vi "Hokuyo URG Series Configure and Acquire Data.vi"() -> ()   [LabVIEW 2011]
doc: "This example shows how to configure the URG to aquire data and then creates a polar graph using the magnitude and direction arrays.\n\nTo use this example with a USB LIDAR on a cRIO target, change the VISA resource name type to USB Raw. See the help for the control for additional information."
uses:
  Public/Initialize-Standard.vi
  Hokuyo URG Series.lvlib
panel:
  in  "Encoding Width":u16(ring)=3 items=["2 Byte"=2, "3 Byte"=3]
  in  "Max (m)":dbl=4.1
  in  "Plot Color":u32(colorbox)=6618880
  in  "Grid Color":u32(colorbox)=16777222
  in  "Protocol":u32(ring)=2 items=["Convert to Latest", "SCIP 1.1", "SCIP 2.0"]
  in  "ID Query?":bool=TRUE
  in  "Cluster Count":dbl=1.0
  in  "Start Point":dbl=-120.0
  in  "End Point":dbl=120.0
  in  "Checksum":bool
  in  "VISA resource name":refnum<visa-resource-name>
  in  "Stop":bool
  in  "polar attributes (hidden)":T1={"maximum"=30000.0, "minimum"=0.0, "clip to min"=FALSE, "log?(F)"=TRUE, "grid color"=6710886, "plot color"=65280, "fmt and prec"={"format"=enum."Decimal", "precision"=0}, "visible section"=8} {"minimum" format="%0.2f"; "maximum" format="%0.2f"}
  out "Data Aquired":picture
  # "(c) 2009 National Instruments.  ALL RIGHTS RESERVED."
  # "Instrument Configuration"
  # "Measurement Configuration"
  # "Plot Display Configuration"
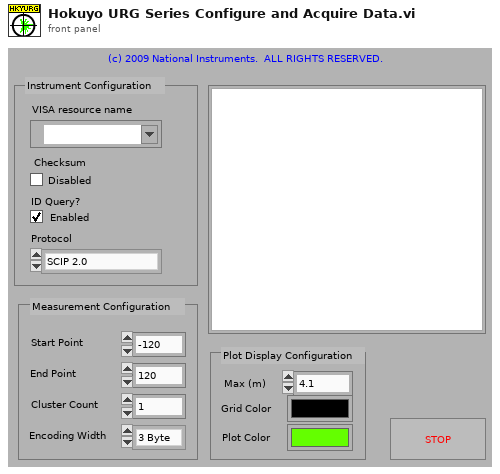
[diagram p1: front panel]
types:
  T1 = cluster{"maximum":dbl, "minimum":dbl, "clip to min":bool, "log?(F)":bool, "grid color":u32, "plot color":u32, "fmt and prec":cluster{"format":enum8{"Decimal", "Scientific", "Engineering", "Binary", "Octal", "Hex"}, "precision":u8}, "visible section":u16}
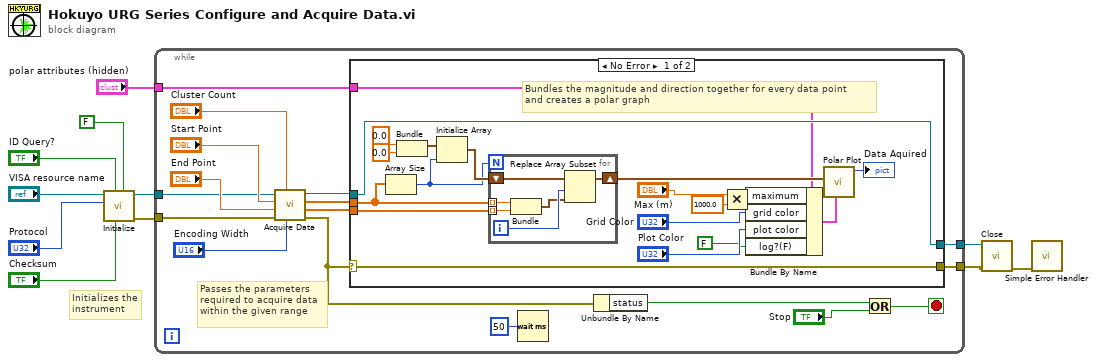
[diagram p0: block diagram]
diagram:
  # "Initializes the instrument"
  n1 = call-poly "Initialize.vi"("Reset? (F: No)"=FALSE ("Reset Instrument (Disabled)"), "Checksum (Disabled)"="Checksum", "ID Query? (Enabled)"="ID Query?", "Protocol (2: SCIP 2.0)"="Protocol", "VISA resource name"="VISA resource name") -> ("error out"=w2:errorcluster, "VISA resource name out"=w3:refnum<visa-resource-name>)  [unwired: 5 in]
  n2 = while {
    tunnel: w3 -> [w16]
    tunnel: [w28] -> w11
    tunnel: [w27] -> w4
    tunnel: w2 -> [w15]
    tunnel: "polar attributes (hidden)" -> [w14]
    stop <- w24 stop-if-true
    # "Passes the parameters\nrequired to acquire data\nwithin the given range"
    n3 = call "Acquire Data.vi"("Data Encoding Width (3 Byte)"="Encoding Width", "Cluster Count (1)"="Cluster Count", "error in (no error)"=w15, "End Point (120°)"="End Point", "Start Point (-120°)"="Start Point", "VISA resource name"=w16) -> ("error out"=w20:errorcluster, "Direction"=w21:dbl[], "Magnitude"=w22:dbl[], "VISA resource name out"=w23:refnum<visa-resource-name>)  [unwired: 2 in]
    n4 = case shown="No Error" w20 {
      selector: w20 -> [w45 w55]
      tunnel: [w45 w55] -> w28
      tunnel: w23 -> [w46 w54]
      tunnel: [w46 w54] -> w27
      tunnel: w22 -> [w40 _]
      tunnel: w21 -> [w39 _]
      tunnel: w14 -> [w35 _]
      frame No Error {
        # "Bundles the magnitude and direction together for every data point\nand creates a polar graph"
        n5 = Array Size(array=w40) -> (size(s)=w38:i32)
        n6 = Bundle(0.0, 0.0) -> (w42:cluster{dbl, dbl})  [unwired: 1 in]
        n7 = Initialize Array(w42, w38) -> (w41:cluster{dbl, dbl}[])
        n8 = for {
          N: w38 -> [_]
          shift-right: [w49] -> w37
          shift-left: w41 -> [w50]
          tunnel: w40 -> [w53] mode=indexing
          tunnel: w39 -> [w52] mode=indexing
          i -> [w51]
          n9 = Bundle(w53, w52) -> (w48:cluster{dbl, dbl})  [unwired: 1 in]
          n10 = Replace Array Subset(array=w50, new element=w48, index=w51) -> (w49:cluster{dbl, dbl}[])
        }
        n11 = Multiply(x="Max (m)", y=1000.0) -> (x*y=w31:dbl)
        n12 = Bundle By Name(cluster=w35, "maximum"=w31, "grid color"="Grid Color", "plot color"="Plot Color", "log?(F)"=FALSE) -> (w36:T1)
        n13 = call <vilib>:"Polar Plot.vi"("polar attributes"=w36, "data array [mag, phase (deg)]"=w37) -> ("new picture"=→"Data Aquired":picture)  [unwired: 9 in]
      }
      frame Error {
      }
    }
    n14 = Wait (ms)(milliseconds to wait=u32 50) -> ()  [unwired: 1 out]
    n15 = Unbundle By Name(w20) -> ("status"=w26:bool)
    n16 = Or(x=w26, y="Stop") -> (x .or. y?=w24:bool)
  }
  n17 = call "Close.vi"("error in (no error)"=w11, "VISA resource name"=w4) -> ("error out"=w8:errorcluster)  [unwired: 9 in]
  n18 = call <vilib>:"Simple Error Handler.vi"("error in (no error)"=w8) -> ()  [unwired: 4 in, 5 out]
